vi "DVR LV2.vi"(0 "Data Value Refnum In":refnum<data-value>, 11 "error in (no error)":errorcluster, 13 "Operation":T1) -> (4 "Data Value Refnum Out":refnum<data-value>, 15 "error out":errorcluster)   [LabVIEW 2023]
doc: "This VI is a functional global that holds the reference of the DVR and writes and read based on the user selection."
uses:
  Controls/Operation.ctl
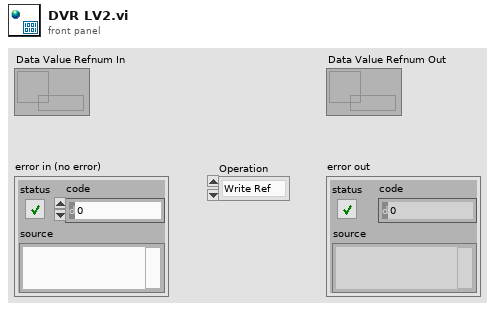
[diagram p1: front panel]
types:
  T1 = typedef "Operation.ctl" = enum16{"Write Ref", "Read Ref"}
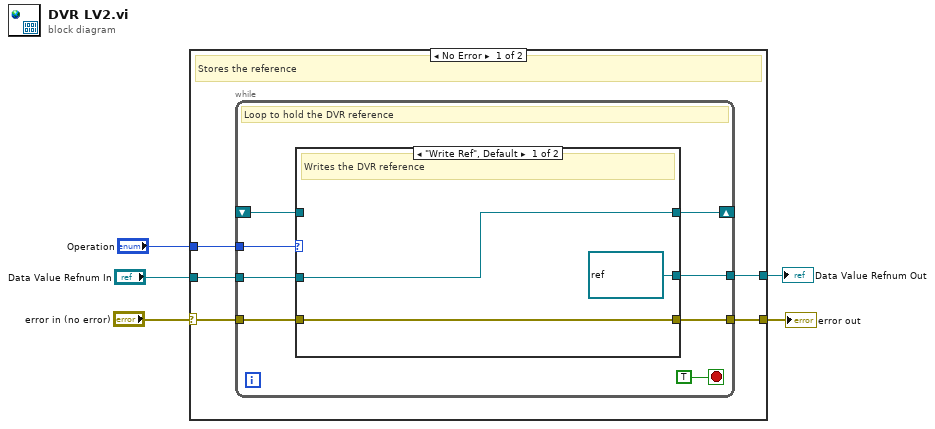
[diagram p0: block diagram]
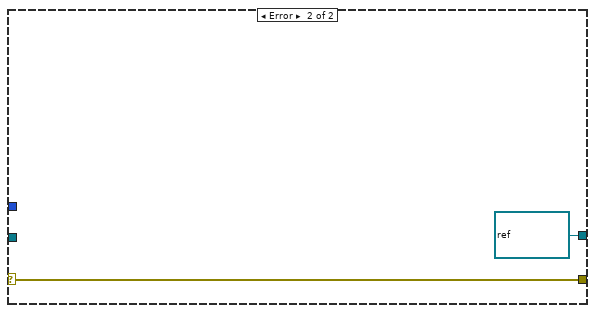
[diagram p3: hidden frame]
diagram:
  n1 = case shown="No Error" "error in (no error)" {
    selector: "error in (no error)" -> [w7 w25]
    tunnel: "Operation" -> [w10 _]
    tunnel: "Data Value Refnum In" -> [w9 _]
    tunnel: [w8 refnum<data-value> refnum ("Data Value Refnum In")] -> w3
    tunnel: [w6 w25] -> w1
    frame No Error {
      # "Stores the reference"
      n2 = while {
        tunnel: w10 -> [w17]
        tunnel: w9 -> [w16]
        shift-right: [w15] -> _
        shift-left: _ -> [w14]
        tunnel: [w13] -> w8
        tunnel: w7 -> [w12]
        tunnel: [w11] -> w6
        stop <- TRUE stop-if-true
        # "Loop to hold the DVR reference"
        n3 = case shown="\"Write Ref\", Default" w17 {
          tunnel: w16 -> [w21 _]
          tunnel: [w21 w23] -> w15
          tunnel: w14 -> [_ w23]
          tunnel: [refnum<data-value> refnum ("Data Value Refnum In") w23] -> w13
          tunnel: w12 -> [w20 w22]
          tunnel: [w20 w22] -> w11
          frame "Write Ref", Default {
            # "Writes the DVR reference"
          }
          frame "Read Ref" {
            # "Reads the DVR reference"
          }
        }
      }
    }
    frame Error {
    }
  }
  "Data Value Refnum Out" <- w3
  "error out" <- w1
